vi "Read HW IO Map.vi"(8 "error in (no error)":errorcluster, 11 "Hardware in":refnum<class "Hardware.lvclass">) -> (0 "error out":errorcluster, 2 "Channel Mapping (Device -> Channel)":string[][](array[string]), 3 "Hardware out":refnum<class "Hardware.lvclass">)   [LabVIEW 2026, in "Hardware.lvlib" / "Hardware.lvclass"]
uses:
  Hardware.lvclass
  Hardware.lvclass/Hardware.ctl
  HW Config/HW Configuration.lvclass/HW Configuration.ctl
  Accessors/Read HW Config Class.vi
  HW Config/Read IO Mapping.vi
  HW Config/HW Configuration.lvclass
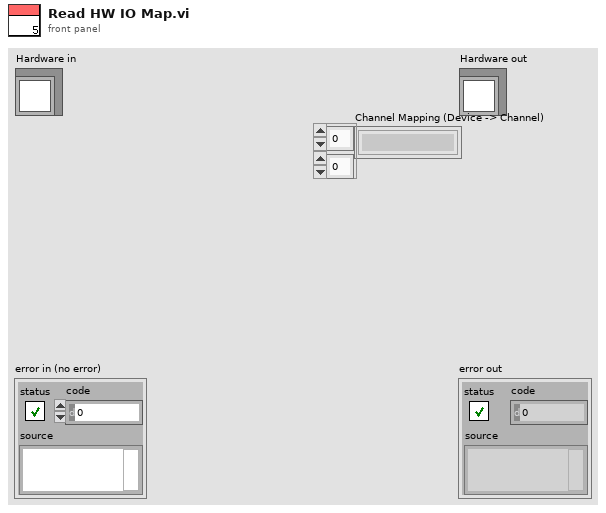
[diagram p1: front panel]
types:
  T1 = cluster{"Device Name":string, "Channel Mapping (Device -> Channel)":string[][]}
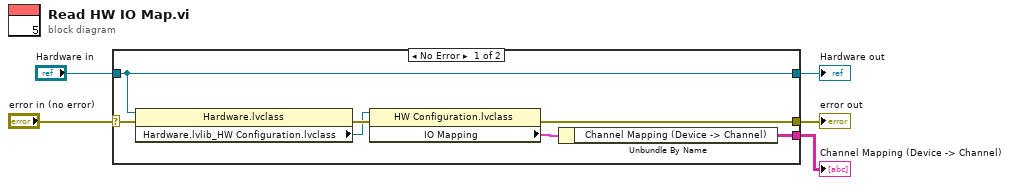
[diagram p0: block diagram]
diagram:
  n1 = case shown="No Error" "error in (no error)" {
    selector: "error in (no error)" -> [w10 w14]
    tunnel: [w8 w14] -> w4
    tunnel: [w11 w13] -> w3
    tunnel: "Hardware in" -> [w11 w13]
    tunnel: [w7 _] -> w2
    frame No Error {
      n2 = property class="Hardware.lvclass"(reference=w11, error in=w10) -> (error out=w9:errorcluster, "Hardware.lvlib_HW Configuration.lvclass"=w6:refnum<class "HW Configuration.lvclass">)  [unwired: 1 out]
      n3 = property class="HW Configuration.lvclass"(reference=w6, error in=w9) -> (error out=w8:errorcluster, "IO Mapping"=w12:T1)  [unwired: 1 out]
      n4 = Unbundle By Name(w12) -> ("Channel Mapping (Device -> Channel)"=w7:string[][])
    }
    frame Error {
    }
  }
  "error out" <- w4
  "Hardware out" <- w3
  "Channel Mapping (Device -> Channel)" <- w2
